vi "Calcul Factor Time.vi"(6 "Accurate Iteration in":i32, 11 "Collision in":refnum<class "Collision.lvclass">) -> (3 "Collision out":refnum<class "Collision.lvclass">)   [LabVIEW 2024, in "Collision.lvclass"]
doc: "MIT Licence\nCopyright (c) 2024 David Grollier"
uses:
  Collision.lvclass
  Collision.lvclass/Collision.ctl
  Game Componants/Game Board Component/Movable/Movable.lvclass
  Game Componants/Game Board Component/Movable/Movable.lvclass/Movable.ctl
panel:
  out "Numeric":dbl
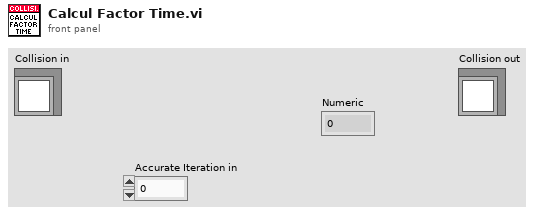
[diagram p1: front panel]
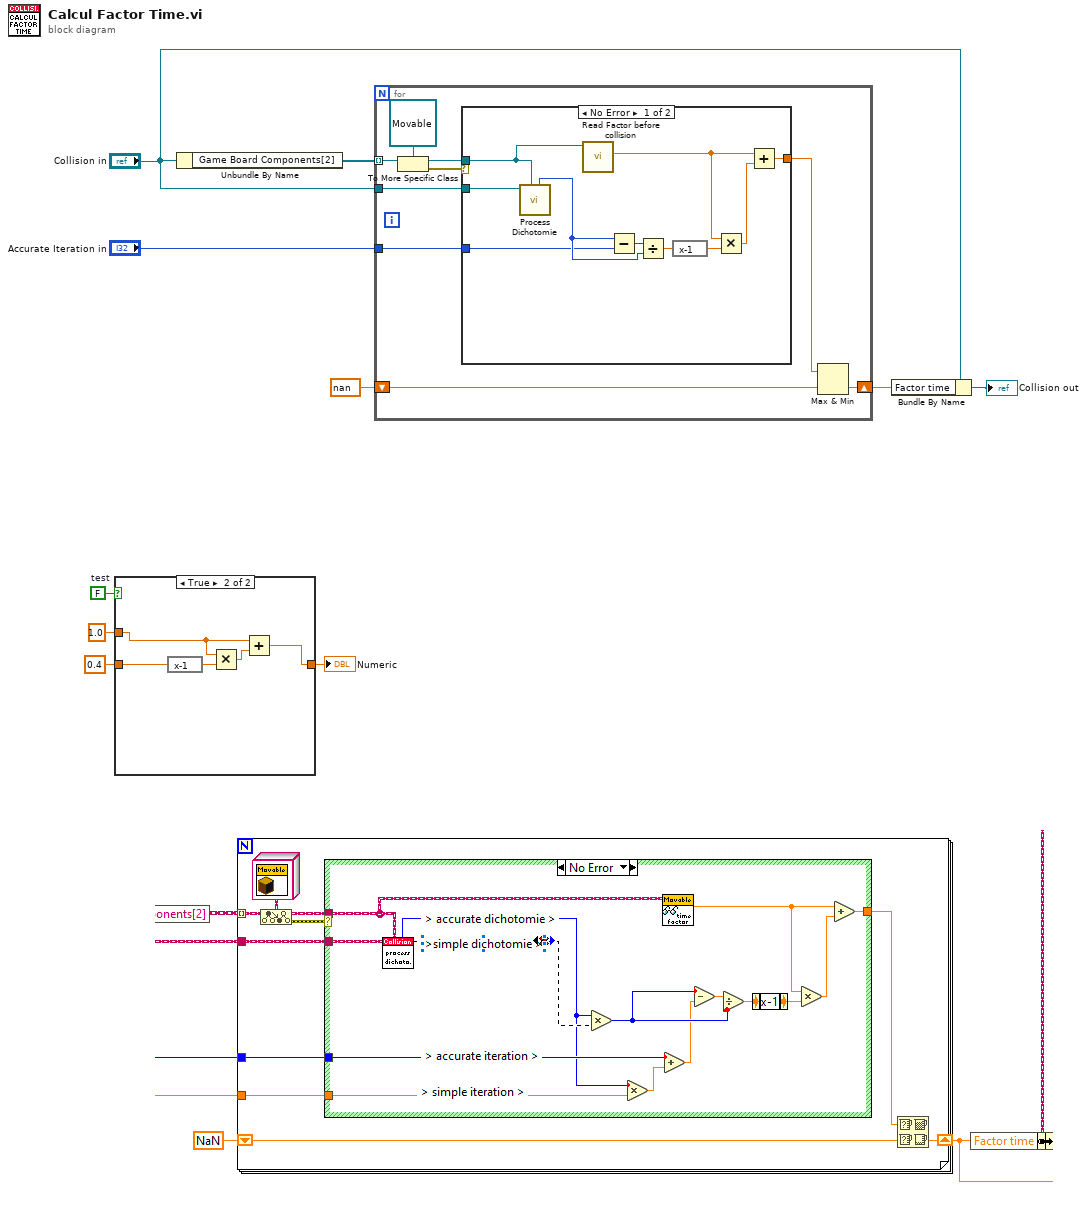
[diagram p0: block diagram]
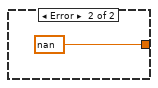
[diagram p3: hidden frame]
diagram:
  w4 = FALSE  # test
  n1 = case shown="True" w4 {
    tunnel: 0.4 -> [w11 w16]
    tunnel: [w11 w13] -> w3
    tunnel: 1.0 ("Factor before collision") -> [_ w12]
    frame False {
    }
    frame True {
      n2 = expression code="x-1"(w16) -> (w15:dbl)
      n3 = Multiply(x=w12, y=w15) -> (x*y=w14:dbl)
      n4 = Add(x=w12, y=w14) -> (x+y=w13:dbl)
    }
  }
  "Numeric" <- w3
  n5 = Unbundle By Name("Collision in") -> ("Game Board Components[2]"=w10:refnum<class "Game Board Component.lvclass">[])
  n6 = for {
    tunnel: w10 -> [w24] mode=indexing
    tunnel: "Collision in" -> [w21]
    tunnel: "Accurate Iteration in" -> [w20]
    shift-right: [w18] -> w6
    shift-left: nan -> [w17]
    n7 = To More Specific Class(target class=refnum<class "Movable.lvclass"> refnum ("Movable.lvclass"), reference=w24) -> (specific class reference=w22:refnum<class "Movable.lvclass">, error out=w23:errorcluster)  [unwired: 1 in]
    n8 = case shown="No Error" w23 {
      tunnel: w22 -> [w31 _]
      tunnel: w21 -> [w35 _]
      tunnel: w20 -> [w32 _]
      tunnel: [w29 nan] -> w19
      frame No Error {
        n9 = call "Process Dichotomie.vi"("Movable in"=w31, "Collision in"=w35) -> ("Dichotomie out"=w33:i32)  [unwired: 8 in, 1 out]
        n10 = call "Read Factor before collision.vi"("Movable in"=w31) -> ("Factor before collision"=w28:dbl)  [unwired: 10 in]
        n11 = Subtract(x=w33, y=w32) -> (x-y=w34:i32)
        n12 = Divide(x=w34, y=w33) -> (x/y=w30:dbl)
        n13 = expression code="x-1"(w30) -> (w26:dbl)
        n14 = Multiply(x=w28, y=w26) -> (x*y=w27:dbl)
        n15 = Add(x=w28, y=w27) -> (x+y=w29:dbl)
      }
      frame Error {
      }
    }
    n16 = Max & Min(x=w19, y=w17) -> (min(x,y)=w18:dbl)  [unwired: 1 out]
  }
  n17 = Bundle By Name(cluster="Collision in", "Factor time"=w6) -> (→"Collision out":refnum<class "Collision.lvclass">)
